vi "DB Tools Type and Dir to ADO.vi"(2 "direction":T1, 3 "data type":T2) -> (0 "ADO direction":u16(ring) items=["adParamUnknown", "adParamInput", "adParamOutput", "adParamInputOutput", "adParamReturnValue"], 1 "ADO type":u16(ring) items=["adEmpty"=0, "adTinyInt"=16, "adSmallInt"=2, "adInteger"=3, "adBigInt"=20, "adUnsignedTinyInt"=17, "adUnsignedSmallInt"=18, "adUnsignedInt"=19, "adUnsignedBigInt"=21, "adSingle"=4, "adDouble"=5, "adCurrency"=6, "adDecimal"=14, "adNumeric"=131, "adBoolean"=11, "adError"=10, "adUserDefined"=132, "adVariant"=12, "adIDispatch"=9, "adIUnknown"=13, "adGUID"=72, "adDate"=7, "adDBDate"=133, "adDBTime"=134, "adDBTimeStamp"=135, "adBSTR"=8, "adChar"=129, "adVarChar"=200, "adLongVarChar"=201, "adWChar"=130, "adVarWChar"=202, "adLongVarWChar"=203, "adBinary"=128, "adVarBinary"=204, "adLongVarBinary"=205, "adChapter"=136, "adFileTime"=64, "adDBFileTime"=137, "adPropVariant"=138, "adVarNumeric"=139])   [LabVIEW 2012, in "NI_Database_API_64.lvlib"]
doc: "Takes the various data types and parameter directions supported by the Database Tools and converts them to the correct parameters used by ADO."
uses:
  NI_Database_API_64.lvlib
  DB Tools DataTypes.ctl
  DB Tools Parameter Dir.ctl
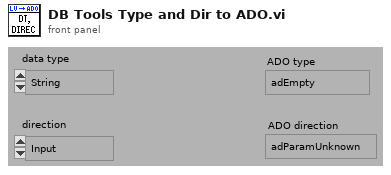
[diagram p1: front panel]
types:
  T1 = typedef "NI_Database_API_64.lvlib/DB Tools Parameter Dir.ctl" = enum32{"Input", "Output", "Input/Output", "Return Value"}
  T2 = typedef "NI_Database_API_64.lvlib/DB Tools DataTypes.ctl" = enum16{"String", "Long (I32)", "Single (SGL)", "Double (DBL)", "Date/Time", "Binary"}
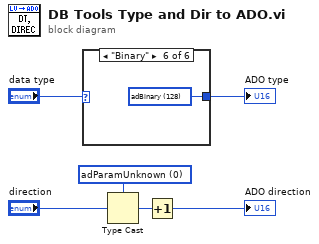
[diagram p0: block diagram]
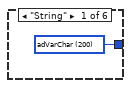
[diagram p2: hidden frame]
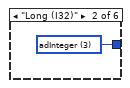
[diagram p3: hidden frame]
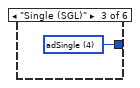
[diagram p4: hidden frame]
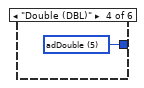
[diagram p5: hidden frame]
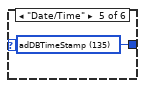
[diagram p6: hidden frame]
diagram:
  w4 = 0 items=["adParamUnknown", "adParamInput", "adParamOutput", "adParamInputOutput", "adParamReturnValue"] ("Direction")
  n1 = case shown="\"Binary\"" "data type" {
    tunnel: [w7 w8 w9 w10 w11 w12] -> w1
    frame "String" {
      w7 = 200 items=["adEmpty"=0, "adTinyInt"=16, "adSmallInt"=2, "adInteger"=3, "adBigInt"=20, "adUnsignedTinyInt"=17, "adUnsignedSmallInt"=18, "adUnsignedInt"=19, "adUnsignedBigInt"=21, "adSingle"=4, "adDouble"=5, "adCurrency"=6, "adDecimal"=14, "adNumeric"=131, "adBoolean"=11, "adError"=10, "adUserDefined"=132, "adVariant"=12, "adIDispatch"=9, "adIUnknown"=13, "adGUID"=72, "adDate"=7, "adDBDate"=133, "adDBTime"=134, "adDBTimeStamp"=135, "adBSTR"=8, "adChar"=129, "adVarChar"=200, "adLongVarChar"=201, "adWChar"=130, "adVarWChar"=202, "adLongVarWChar"=203, "adBinary"=128, "adVarBinary"=204, "adLongVarBinary"=205, "adChapter"=136, "adFileTime"=64, "adDBFileTime"=137, "adPropVariant"=138, "adVarNumeric"=139] ("Type")
    }
    frame "Long (I32)" {
      w8 = 3 items=["adEmpty"=0, "adTinyInt"=16, "adSmallInt"=2, "adInteger"=3, "adBigInt"=20, "adUnsignedTinyInt"=17, "adUnsignedSmallInt"=18, "adUnsignedInt"=19, "adUnsignedBigInt"=21, "adSingle"=4, "adDouble"=5, "adCurrency"=6, "adDecimal"=14, "adNumeric"=131, "adBoolean"=11, "adError"=10, "adUserDefined"=132, "adVariant"=12, "adIDispatch"=9, "adIUnknown"=13, "adGUID"=72, "adDate"=7, "adDBDate"=133, "adDBTime"=134, "adDBTimeStamp"=135, "adBSTR"=8, "adChar"=129, "adVarChar"=200, "adLongVarChar"=201, "adWChar"=130, "adVarWChar"=202, "adLongVarWChar"=203, "adBinary"=128, "adVarBinary"=204, "adLongVarBinary"=205, "adChapter"=136, "adFileTime"=64, "adDBFileTime"=137, "adPropVariant"=138, "adVarNumeric"=139] ("Type")
    }
    frame "Single (SGL)" {
      w9 = 4 items=["adEmpty"=0, "adTinyInt"=16, "adSmallInt"=2, "adInteger"=3, "adBigInt"=20, "adUnsignedTinyInt"=17, "adUnsignedSmallInt"=18, "adUnsignedInt"=19, "adUnsignedBigInt"=21, "adSingle"=4, "adDouble"=5, "adCurrency"=6, "adDecimal"=14, "adNumeric"=131, "adBoolean"=11, "adError"=10, "adUserDefined"=132, "adVariant"=12, "adIDispatch"=9, "adIUnknown"=13, "adGUID"=72, "adDate"=7, "adDBDate"=133, "adDBTime"=134, "adDBTimeStamp"=135, "adBSTR"=8, "adChar"=129, "adVarChar"=200, "adLongVarChar"=201, "adWChar"=130, "adVarWChar"=202, "adLongVarWChar"=203, "adBinary"=128, "adVarBinary"=204, "adLongVarBinary"=205, "adChapter"=136, "adFileTime"=64, "adDBFileTime"=137, "adPropVariant"=138, "adVarNumeric"=139] ("Type")
    }
    frame "Double (DBL)" {
      w10 = 5 items=["adEmpty"=0, "adTinyInt"=16, "adSmallInt"=2, "adInteger"=3, "adBigInt"=20, "adUnsignedTinyInt"=17, "adUnsignedSmallInt"=18, "adUnsignedInt"=19, "adUnsignedBigInt"=21, "adSingle"=4, "adDouble"=5, "adCurrency"=6, "adDecimal"=14, "adNumeric"=131, "adBoolean"=11, "adError"=10, "adUserDefined"=132, "adVariant"=12, "adIDispatch"=9, "adIUnknown"=13, "adGUID"=72, "adDate"=7, "adDBDate"=133, "adDBTime"=134, "adDBTimeStamp"=135, "adBSTR"=8, "adChar"=129, "adVarChar"=200, "adLongVarChar"=201, "adWChar"=130, "adVarWChar"=202, "adLongVarWChar"=203, "adBinary"=128, "adVarBinary"=204, "adLongVarBinary"=205, "adChapter"=136, "adFileTime"=64, "adDBFileTime"=137, "adPropVariant"=138, "adVarNumeric"=139] ("Type")
    }
    frame "Date/Time" {
      w11 = 135 items=["adEmpty"=0, "adTinyInt"=16, "adSmallInt"=2, "adInteger"=3, "adBigInt"=20, "adUnsignedTinyInt"=17, "adUnsignedSmallInt"=18, "adUnsignedInt"=19, "adUnsignedBigInt"=21, "adSingle"=4, "adDouble"=5, "adCurrency"=6, "adDecimal"=14, "adNumeric"=131, "adBoolean"=11, "adError"=10, "adUserDefined"=132, "adVariant"=12, "adIDispatch"=9, "adIUnknown"=13, "adGUID"=72, "adDate"=7, "adDBDate"=133, "adDBTime"=134, "adDBTimeStamp"=135, "adBSTR"=8, "adChar"=129, "adVarChar"=200, "adLongVarChar"=201, "adWChar"=130, "adVarWChar"=202, "adLongVarWChar"=203, "adBinary"=128, "adVarBinary"=204, "adLongVarBinary"=205, "adChapter"=136, "adFileTime"=64, "adDBFileTime"=137, "adPropVariant"=138, "adVarNumeric"=139] ("Type")
    }
    frame "Binary" {
      w12 = 128 items=["adEmpty"=0, "adTinyInt"=16, "adSmallInt"=2, "adInteger"=3, "adBigInt"=20, "adUnsignedTinyInt"=17, "adUnsignedSmallInt"=18, "adUnsignedInt"=19, "adUnsignedBigInt"=21, "adSingle"=4, "adDouble"=5, "adCurrency"=6, "adDecimal"=14, "adNumeric"=131, "adBoolean"=11, "adError"=10, "adUserDefined"=132, "adVariant"=12, "adIDispatch"=9, "adIUnknown"=13, "adGUID"=72, "adDate"=7, "adDBDate"=133, "adDBTime"=134, "adDBTimeStamp"=135, "adBSTR"=8, "adChar"=129, "adVarChar"=200, "adLongVarChar"=201, "adWChar"=130, "adVarWChar"=202, "adLongVarWChar"=203, "adBinary"=128, "adVarBinary"=204, "adLongVarBinary"=205, "adChapter"=136, "adFileTime"=64, "adDBFileTime"=137, "adPropVariant"=138, "adVarNumeric"=139] ("Type")
    }
  }
  "ADO type" <- w1
  n2 = Type Cast(type=w4, x="direction") -> (*(type *) &x=w5:i32)
  n3 = Increment(x=w5) -> (x+1=→"ADO direction":i32)
